vi "Send command Set Port.vi"(7 "Marca":string, 8 "error in (no error)":errorcluster, 9 "Valor HEX":string, 10 "Puerto":string, 11 "Arduino in":refnum<class "Arduino.lvclass">) -> (0 "error out":errorcluster, 1 "Command":string, 2 "Expected response":string, 3 "Arduino out":refnum<class "Arduino.lvclass">)   [LabVIEW 2020, in "Arduino.lvclass"]
uses:
  Arduino.lvclass
  Arduino.lvclass/Arduino.ctl
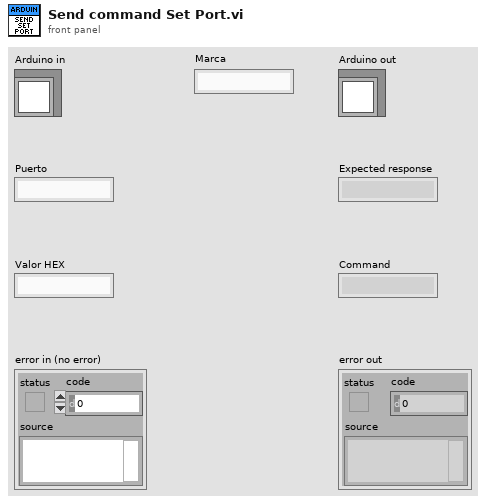
[diagram p1: front panel]
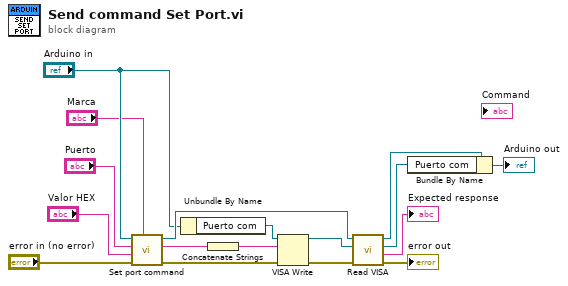
[diagram p0: block diagram]
diagram:
  n1 = call-dynamic "Set port command.vi"("Marca"="Marca", "error in (no error)"="error in (no error)", "Valor HEX"="Valor HEX", "Puerto"="Puerto", "Serial Device in"="Arduino in") -> ("error out"=w16:errorcluster, "Command"=w13:string, "Serial Device out"=w15:refnum<class "Arduino.lvclass">)  [unwired: 3 in, 1 out]
  n2 = Unbundle By Name("Arduino in") -> ("Puerto com"=w12:refnum<visa-resource-name>)
  n3 = Concatenate Strings(w13) -> (w14:string)
  n4 = VISA Write(VISA resource name=w12, write buffer=w14, error in (no error)=w16) -> (VISA resource name out=w11:refnum<visa-resource-name>, error out=w17:errorcluster)  [unwired: 1 out]
  n5 = call-dynamic "Read VISA.vi"("error in (no error)"=w17, "VISA Refnum in"=w11, "Serial Device in"=w15) -> ("error out"=→"error out":errorcluster, "Serial Response"=→"Expected response":string, "VISA resource name out"=w9:refnum<visa-resource-name>, "Serial Device out"=w10:refnum<class "Arduino.lvclass">)  [unwired: 5 in]
  n6 = Bundle By Name(cluster=w10, "Puerto com"=w9) -> (→"Arduino out":refnum<class "Arduino.lvclass">)
